vi "FRCts20_Backend_BuildAppXMLPath.vi"(8 "error in (no error)":errorcluster) -> (0 "error out":errorcluster, 2 "Path Out":path)   [LabVIEW 2014, in "FRCts20_Backend_Engine.lvlib"]
doc: "Generates path to public data folder on computer."
uses:
  FRCts20_Backend_Engine.lvlib
  <vilib>/Utility/sysdir.llb/System Directory Type.ctl
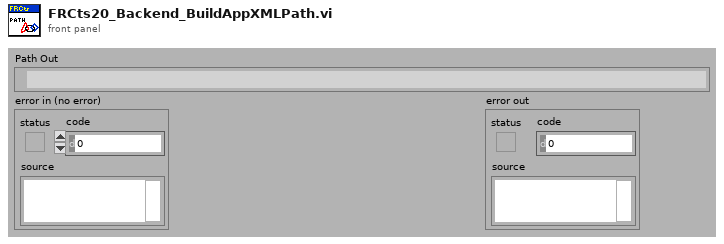
[diagram p1: front panel]
types:
  T1 = typedef "System Directory Type.ctl" = i32
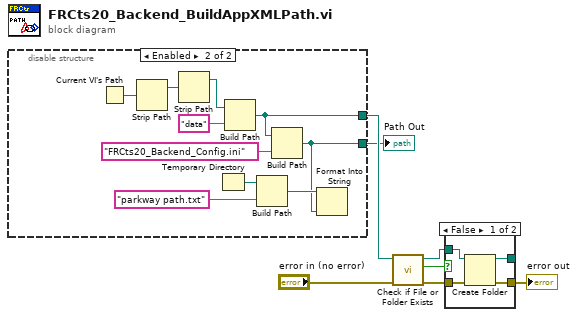
[diagram p0: block diagram]
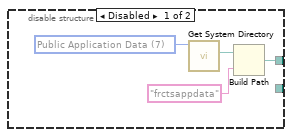
[diagram p2: hidden frame]
diagram:
  n1 = disable-structure shown="Enabled" {
    disable-tunnel: [w8 w13] -> w2
    disable-tunnel: [_ w12] -> w1
    frame Disabled {
      w11 = T1 7 items=["User Home"=0, "User Desktop"=1, "User Documents"=2, "User Application Data"=3, "User Preferences"=4, "User Temporary"=5, "Public Documents"=6, "Public Application Data"=7, "Public Preferences"=8, "Public Cache"=13, "System Core Libraries"=9, "System Installed Libraries"=10, "Application Files"=11, "Boot Volume Root"=12] ("system directory type")
      n2 = call <vilib>:"Get System Directory.vi"("system directory type"=w11) -> ("system directory"=w9:path)  [unwired: 10 in]
      n3 = Build Path(base path=w9, name or relative path="frctsappdata") -> (appended path=w8:path)
    }
    frame Enabled {
      n4 = Current VI's Path() -> (path=w21:path)
      n5 = Strip Path(path=w21) -> (stripped path=w17:path)  [unwired: 1 out]
      n6 = Strip Path(path=w17) -> (stripped path=w16:path)  [unwired: 1 out]
      n7 = Temporary Directory() -> (w20:path)
      n8 = Build Path(base path=w16, name or relative path="data") -> (appended path=w13:path)
      n9 = Build Path(base path=w20, name or relative path="parkway path.txt") -> (appended path=w18:path)
      n10 = Build Path(base path=w13, name or relative path="FRCts20_Backend_Config.ini") -> (appended path=w12:path)
      n11 = Format Into String(initial string=w18, w12) -> ()  [unwired: 2 in, 2 out]
    }
  }
  "Path Out" <- w1
  n12 = call <vilib>:"Check if File or Folder Exists.vi"("error in (no error)"="error in (no error)", "path"=w2) -> ("error out"=w5:errorcluster, "file or folder exists?"=w7:bool, "dup path"=w6:path)  [unwired: 7 in]
  n13 = case shown="False" w7 {
    tunnel: w6 -> [w25 w27]
    tunnel: w5 -> [w24 w26]
    tunnel: [w23 w26] -> w3
    tunnel: [w22 w27] -> _
    frame False {
      n14 = Create Folder(path (use dialog)=w25, error in=w24) -> (created path=w22:path, error out=w23:errorcluster)  [unwired: 1 in, 1 out]
    }
    frame True {
    }
  }
  "error out" <- w3
